vi "Argo_Drive.vi"(0 "Speed_Main":dbl=-0.047244094488188976, 1 "Speed_Limit":dbl=0.047244094488188976, 3 "Turning_Limit":dbl=-0.023622047244094488, 4 "Turning_PID_Enable":bool, 5 "PID Gains":T1, 6 "Turning_Main":dbl=-0.007874015748031496, 7 "Auto_Enable":bool, 8 "High_Gear":bool, 9 "Quick_Turn":bool=TRUE, 10 "Turning_Setpoint":dbl, 11 "dt (s)":dbl=10.0 format="%.3f", 14 "Yaw":dbl=654.9580428601698) -> (12 "Left_Motor":dbl format="%.2f", 13 "Right_Motor":dbl format="%.2f")   [LabVIEW 2015]
panel:
  out "Waveform Chart":cluster{"Left_Motor_Sat":dbl, "Output":dbl}(graph)
  in  "Ramp_Rate":dbl=0.2
  in  "High_Turning Y":dbl[](array[numeric])=[-0.4, -0.25, -0.1, 0.0, 0.0, 0.0, 0.1, 0.25, 0.4]
  in  "High_Turning X":dbl[](array[numeric])=[-1.0, -0.75, -0.21, -0.2, 0.0, 0.2, 0.21, 0.75, 1.0]
  in  "Low_Turning Y":dbl[](array[numeric])=[-1.0, -0.4, -0.1, 0.0, 0.0, 0.0, 0.1, 0.4, 1.0]
  in  "Low_Turning X":dbl[](array[numeric])=[-1.0, -0.75, -0.2, -0.19, 0.0, 0.19, 0.2, 0.75, 1.0]
  in  "Auto_Turning Y":dbl[](array[numeric])=[-1.0, -0.003, -0.002, -0.001, 0.0, 0.001, 0.002, 0.003, 1.0]
  in  "Auto_Turning X":dbl[](array[numeric])=[-1.0, -0.75, -0.12, -0.1, 0.0, 0.1, 0.12, 0.75, 1.0]
  in  "Low Speed Y":dbl[](array[numeric])=[-1.0, -0.4, -0.15, 0.0, 0.0, 0.0, 0.15, 0.4, 1.0]
  in  "Low Speed X":dbl[](array[numeric])=[-1.0, -0.75, -0.21, -0.2, 0.0, 0.2, 0.21, 0.75, 1.0]
  in  "High Speed Y":dbl[](array[numeric])=[-0.85, -0.5, -0.15, 0.0, 0.0, 0.0, 0.15, 0.5, 0.85]
  in  "High Speed X":dbl[](array[numeric])=[-1.0, -0.75, -0.11, -0.1, 0.0, 0.1, 0.11, 0.75, 1.0]
  in  "Auto Speed X":dbl[](array[numeric])=[-1.0, -0.75, -0.06, -0.05, 0.0, 0.05, 0.06, 0.75, 1.0]
  in  "Auto Speed Y":dbl[](array[numeric])=[-1.0, -0.4, -0.15, 0.0, 0.0, 0.0, 0.15, 0.4, 1.0]
  out "XY Turning":cluster{"Turning X ":dbl[], "Turning Y":dbl[]}(graph)={"Turning X "=[-1.0, -0.75, -0.2, -0.19, 0.0, 0.19, 0.2, 0.75, 1.0], "Turning Y"=[-1.0, -0.4, -0.1, 0.0, 0.0, 0.0, 0.1, 0.4, 1.0]}
  out "XY Speed":cluster{"Speed X":dbl[], "Speed Y":dbl[]}(graph)={"Speed X"=[-1.0, -0.75, -0.21, -0.2, 0.0, 0.2, 0.21, 0.75, 1.0], "Speed Y"=[-1.0, -0.4, -0.15, 0.0, 0.0, 0.0, 0.15, 0.4, 1.0]}
  in  "Turning Scale":dbl=1.5
  in  "Turning_Hyd_Deadband":dbl=0.75
  in  "Speed_Hyd_Deadband":dbl=0.75
  out "Delta":dbl format="%.2f"
  # "Chessy Drive"
  # "This subystem takes turning and speed controls from a xbox joystick \nand creats left and right motor values"
  # "Tunning"
  # "Inputs"
  # "Test Points"
  # "Ouputs"
  # "Joystick Map (Lookup Table)"
  # "Hyp Cmd Deadband"
  # "Turning Power Mode"
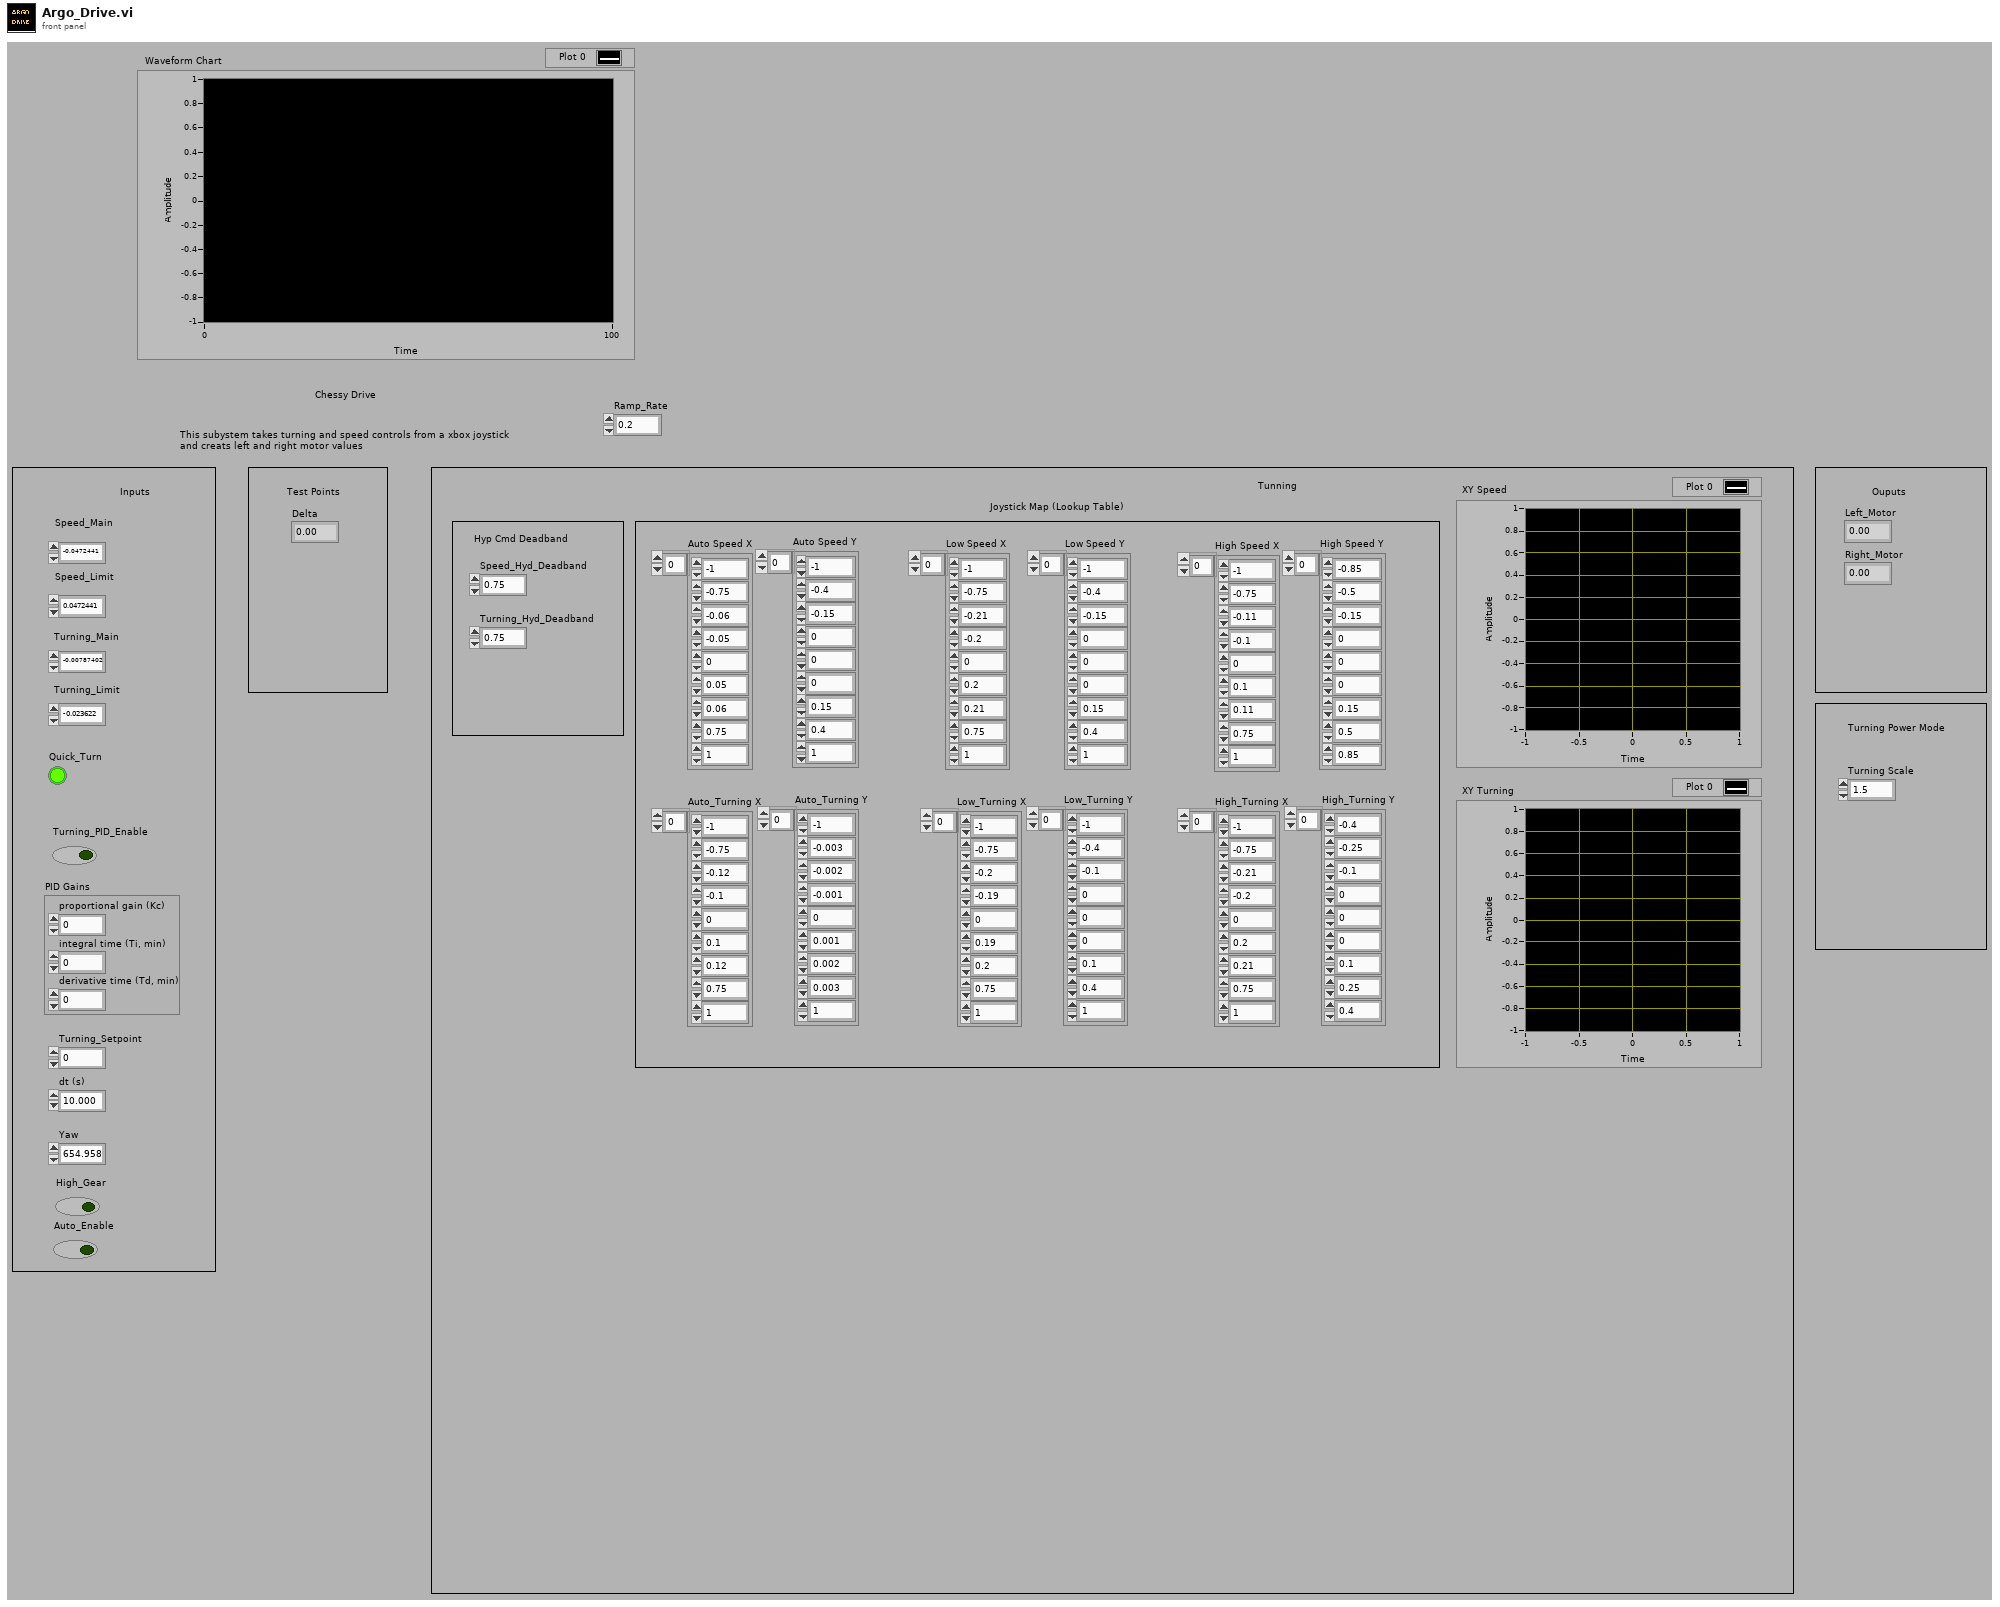
[diagram p1: front panel]
types:
  T1 = cluster{"proportional gain (Kc)":dbl, "integral time (Ti, min)":dbl, "derivative time (Td, min)":dbl}
  T2 = cluster{"Auto_Turning X ":dbl[], "Auto_Turning Y":dbl[]}
  T3 = cluster{"Auto Speed X":dbl[], "Auto Speed Y":dbl[]}
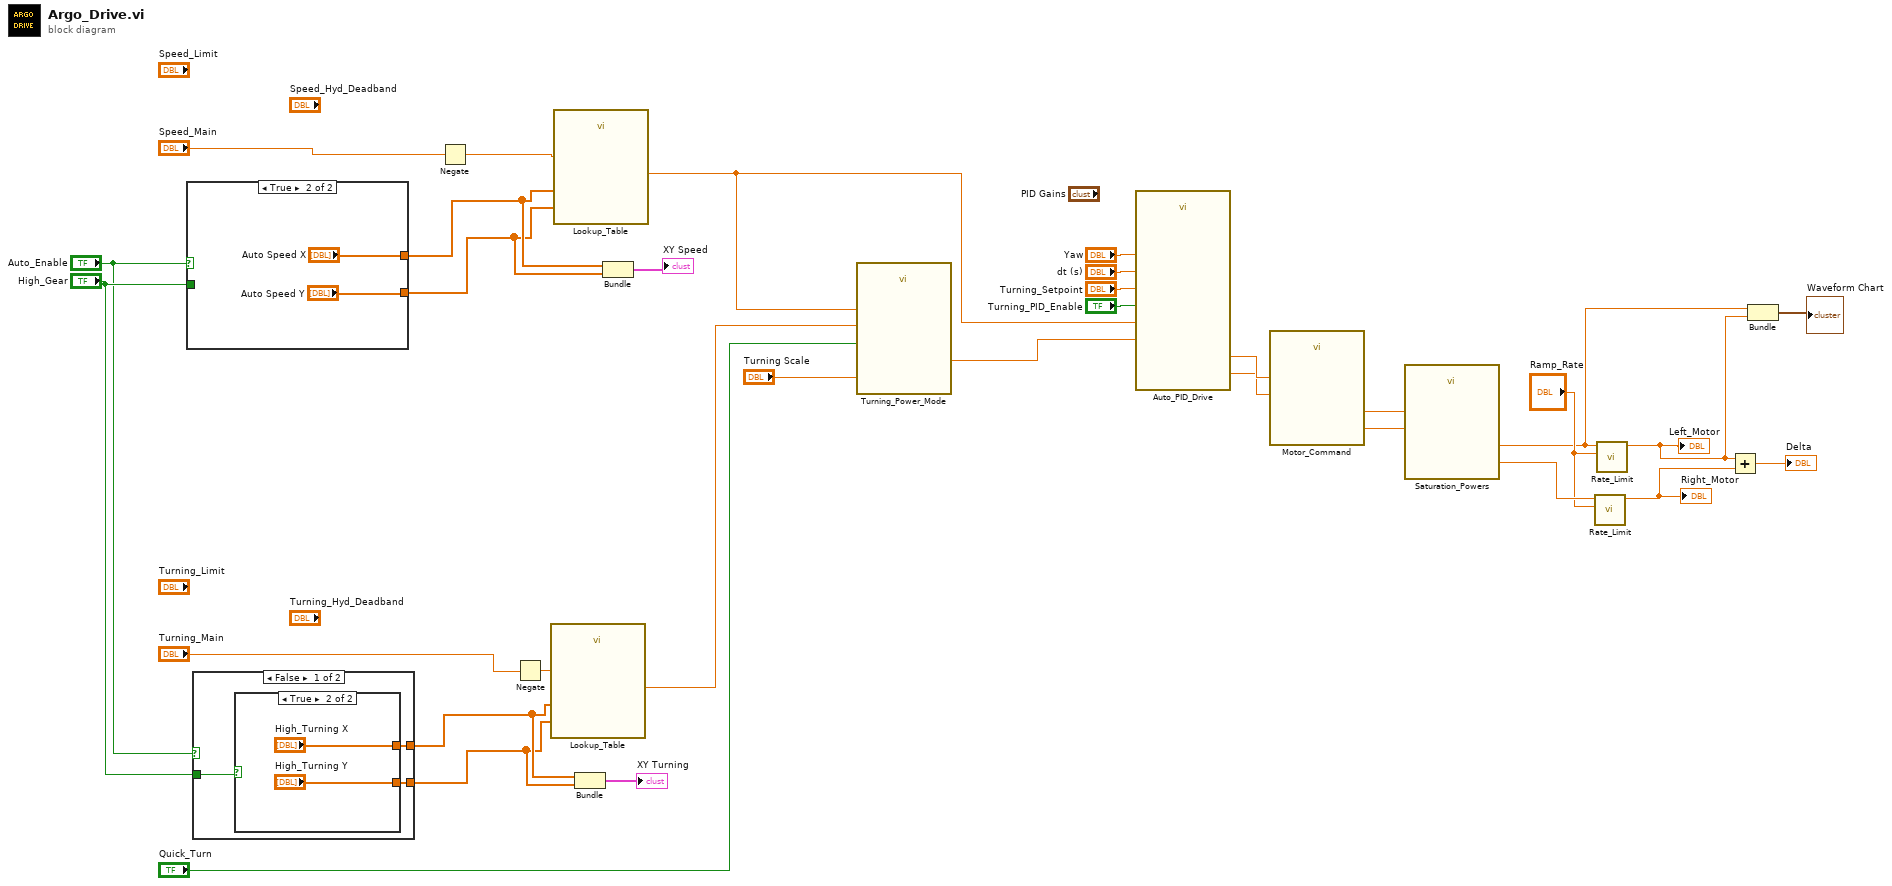
[diagram p0: block diagram]
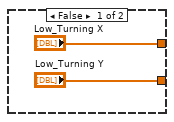
[diagram p2: hidden frame]
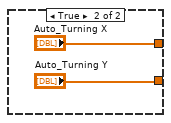
[diagram p3: hidden frame]
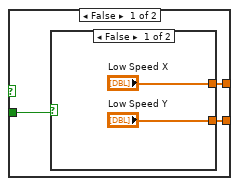
[diagram p4: hidden frame]
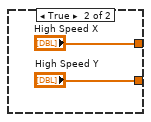
[diagram p5: hidden frame]
diagram:
  n1 = case shown="True" "Auto_Enable" {
    tunnel: "High_Gear" -> [w35 _]
    tunnel: [w34 "Auto Speed X"] -> w17
    tunnel: [w33 "Auto Speed Y"] -> w16
    frame False {
      n2 = case shown="False" w35 {
        tunnel: ["Low Speed X" "High Speed X"] -> w34
        tunnel: ["Low Speed Y" "High Speed Y"] -> w33
        frame False {
        }
        frame True {
        }
      }
    }
    frame True {
    }
  }
  n3 = case shown="False" "Auto_Enable" {
    tunnel: "High_Gear" -> [w44 _]
    tunnel: [w43 "Auto_Turning X"] -> w15
    tunnel: [w42 "Auto_Turning Y"] -> w14
    frame False {
      n4 = case shown="True" w44 {
        tunnel: ["Low_Turning X" "High_Turning X"] -> w43
        tunnel: ["Low_Turning Y" "High_Turning Y"] -> w42
        frame False {
        }
        frame True {
        }
      }
    }
    frame True {
    }
  }
  n5 = Negate(x="Speed_Main") -> (-x=w8:dbl)
  n6 = Negate(x="Turning_Main") -> (-x=w11:dbl)
  n7 = call "Lookup_Table.vi"("Y_Array"=w14, "x_in"=w11, "X_Array"=w15) -> ("y_out"=w25:dbl)  [unwired: 6 in]
  n8 = call "Lookup_Table.vi"("Y_Array"=w16, "x_in"=w8, "X_Array"=w17) -> ("y_out"=w7:dbl)  [unwired: 6 in]
  n9 = Bundle("Auto_Turning X"=w15, "Auto_Turning Y"=w14) -> (→"XY Turning":T2)  [unwired: 1 in]
  n10 = Bundle("Auto Speed X"=w17, "Auto Speed Y"=w16) -> (→"XY Speed":T3)  [unwired: 1 in]
  n11 = call "Turning_Power_Mode.vi"("Turning_Scale"="Turning Scale", "Quick_Turn"="Quick_Turn", "Turning"=w25, "Power"=w7) -> ("Turning_Correction"=w22:dbl)  [unwired: 7 in]
  n12 = call "Auto_PID_Drive.vi"("Turning_PID_Enable"="Turning_PID_Enable", "dt (s)"="dt (s)", "Turning_Setpoint"="Turning_Setpoint", "Yaw"="Yaw", "Turning"=w22, "Power"=w7) -> ("Turning"=w23:dbl, "Power"=w24:dbl)  [unwired: 3 in]
  n13 = call "Motor_Command.vi"("Turning"=w23, "Power"=w24) -> ("Right_Motor"=w31:dbl, "Left_Motor"=w29:dbl)  [unwired: 8 in]
  n14 = call "Saturation_Powers.vi"("Right_Motor"=w31, "Left_Motor"=w29) -> ("Right_Motor_Say"=w6:dbl, "Left_Motor_Sat"=w1:dbl)  [unwired: 8 in]
  n15 = call "Rate_Limit.vi"("Ramp_Rate"="Ramp_Rate", "Input"=w6) -> ("Output"=w4:dbl)  [unwired: 9 in]
  "Right_Motor" <- w4
  n16 = call "Rate_Limit.vi"("Ramp_Rate"="Ramp_Rate", "Input"=w1) -> ("Output"=w2:dbl)  [unwired: 9 in]
  "Left_Motor" <- w2
  n17 = Add(x=w2, y=w4) -> (x+y=→"Delta":dbl)
  n18 = Bundle("Left_Motor_Sat"=w1, "Output"=w2) -> (→"Waveform Chart":cluster{"Left_Motor_Sat":dbl, "Output":dbl})  [unwired: 1 in]
